vi "gjson_UnFlatten.vi"(6 "UnFlattenedData In":string, 8 "error in":errorcluster, 10 "Variant":variant, 11 "JSON String In":string) -> (0 "error out":errorcluster, 2 "UnFlattenData Out":string, 3 "JSON String Out":string)   [LabVIEW 2015, in "Json2Labv.lvlib"]
uses:
  Json2Labv.lvlib
  <vilib>/regexp/Match Regular Expression.xnode
  <vilib>/Utility/VariantDataType/VariantType.lvlib
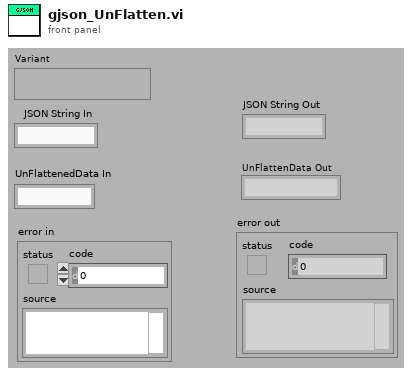
[diagram p1: front panel]
types:
  T1 = typedef "VariantType.lvlib/Type.ctl" = enum8{"Invalid Type", "Void", "I8", "I16", "I32", "I64", "U8", "U16", "U32", "U64", "Single Float", "Double Float", "Extended Float", "Single Complex", "Double Complex", "Extended Complex", "Enum U8", "Enum U16", "Enum U32", "Enum U64", "Single Float With Unit", "Double Float With Unit", "Extended Float With Unit", "Single Complex with Unit", "Double Complex with Unit", "Extended Complex with Unit", "Boolean", "String", "Path", "Picture", "Tag", "Array", "Cluster", "Variant", "LV Variant", "Waveform", "Timestamp", "Digital Waveform", "Digital Data", "ExpressData", "Refnum", "External Data", "VI", "Poly VI", "LabVIEW Class Instance", "Fixed Point"}
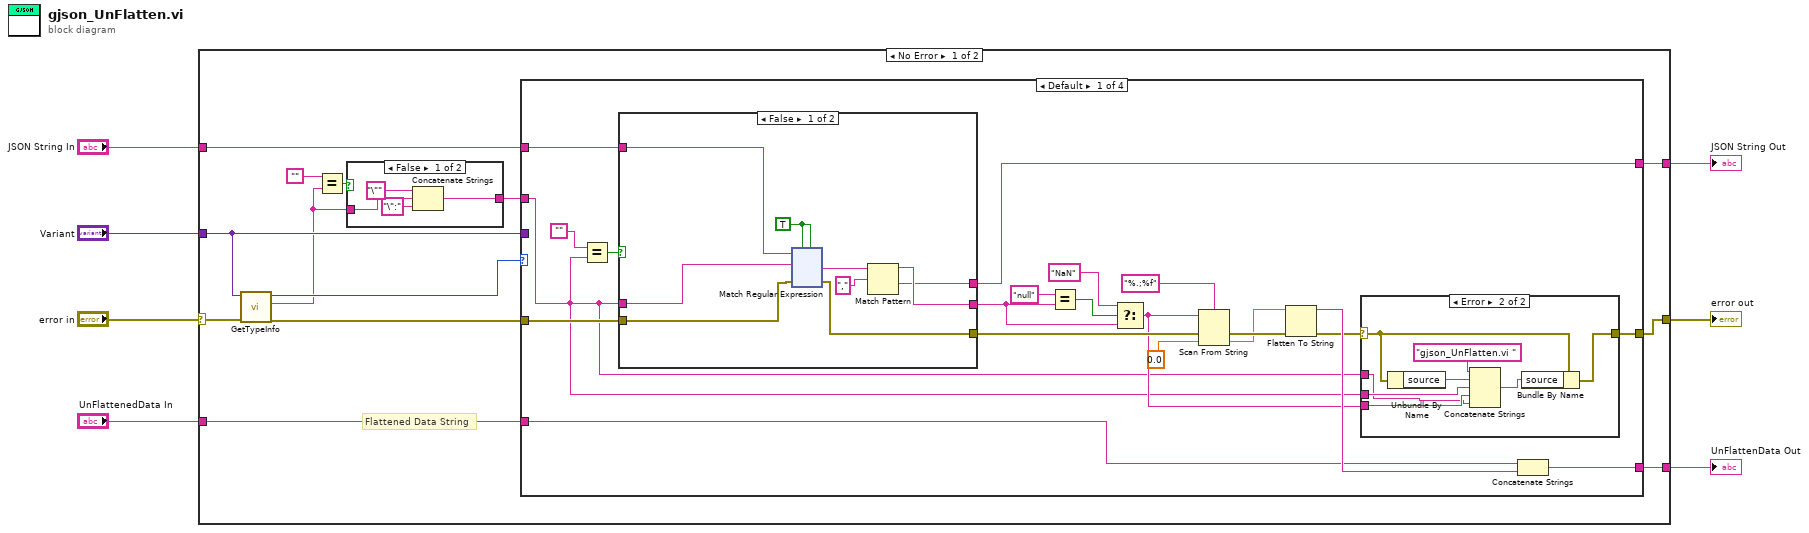
[diagram p0: block diagram]
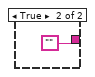
[diagram p2: hidden frame]
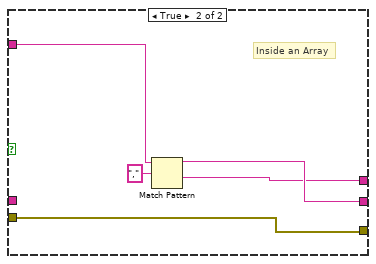
[diagram p4: hidden frame]
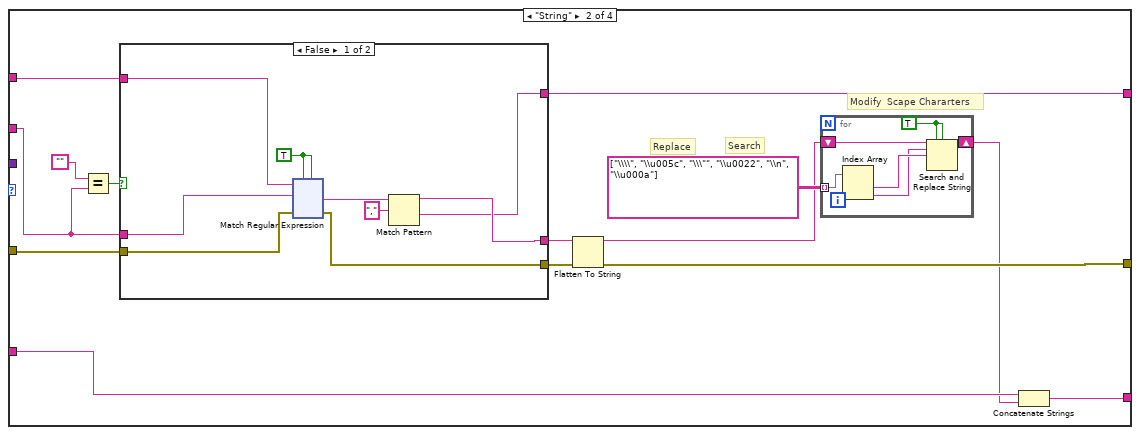
[diagram p5: hidden frame]
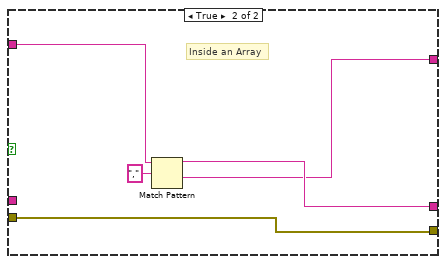
[diagram p6: hidden frame]
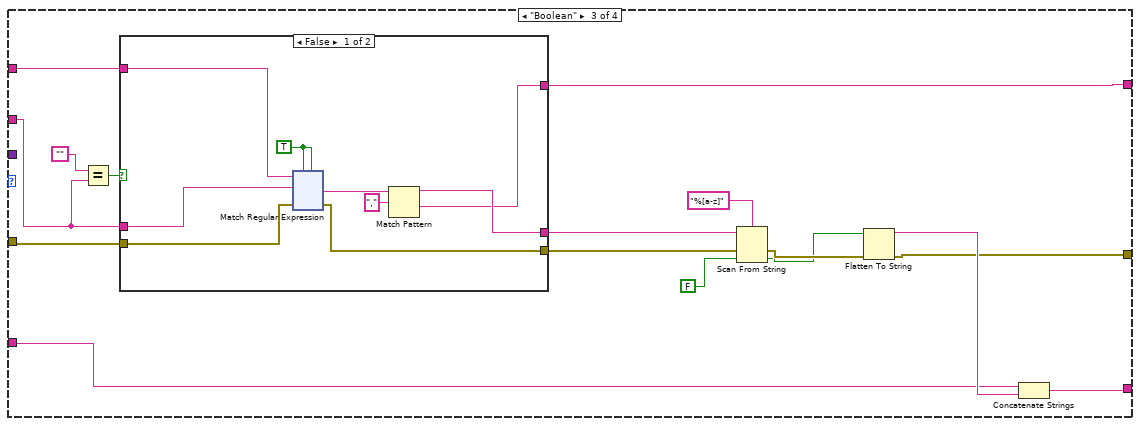
[diagram p7: hidden frame]
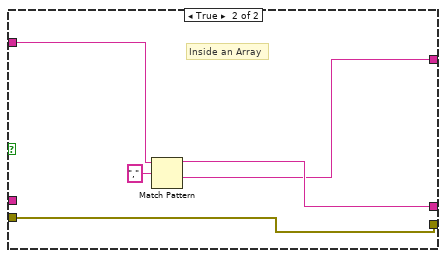
[diagram p8: hidden frame]
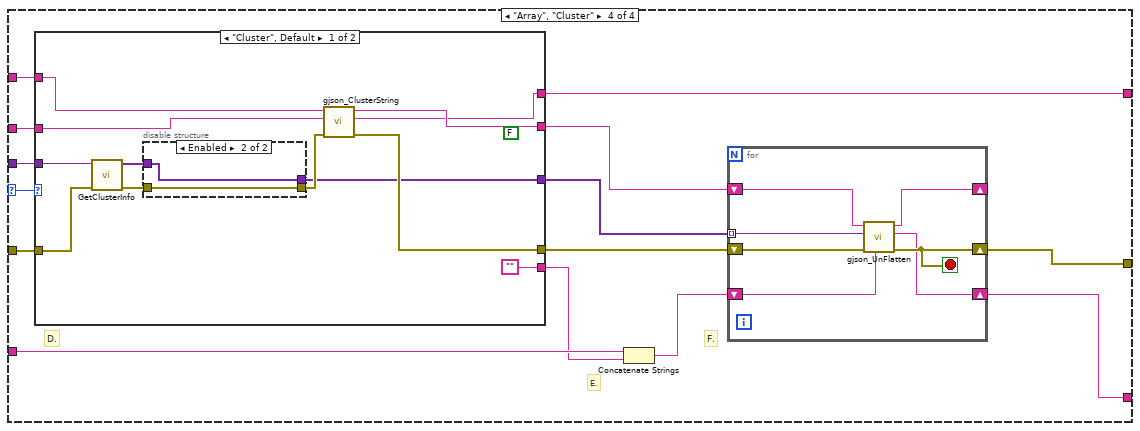
[diagram p9: hidden frame]
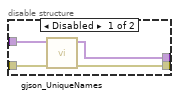
[diagram p10: hidden frame]
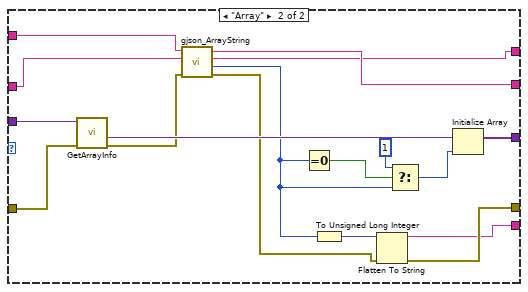
[diagram p11: hidden frame]
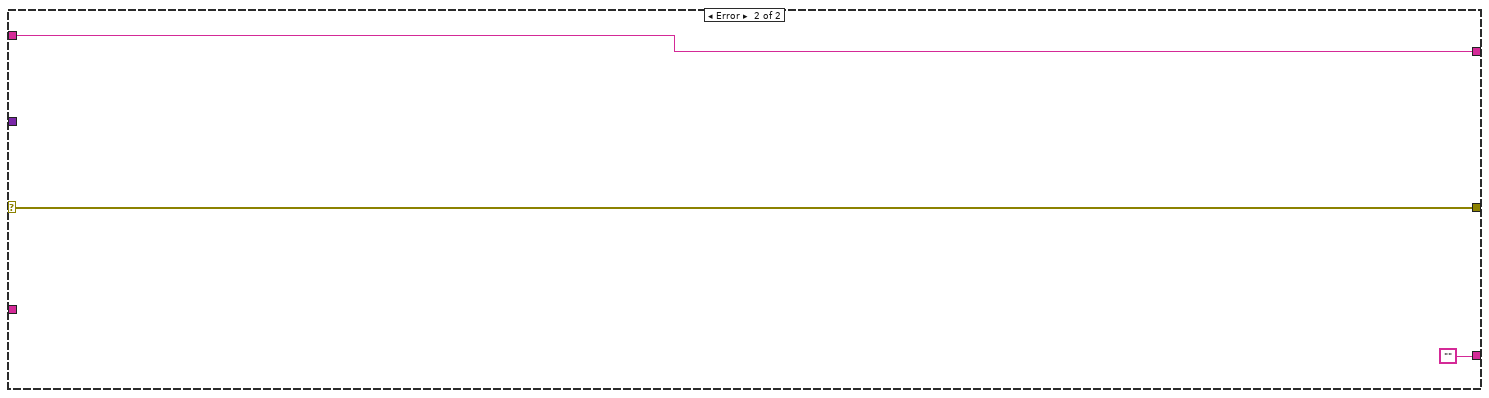
[diagram p12: hidden frame]
diagram:
  n1 = case shown="No Error" "error in" {
    selector: "error in" -> [w18 w525]
    tunnel: [w20 w525] -> w7
    tunnel: [w19 w524] -> w5
    tunnel: "JSON String In" -> [w13 w524]
    tunnel: "Variant" -> [w16 _]
    tunnel: "UnFlattenedData In" -> [w15 _]
    tunnel: [w12 ""] -> w4
    frame No Error {
      # "Flattened Data String"
      n2 = call <vilib>:"GetTypeInfo.vi"("error in (no error)"=w18, "Variant"=w16) -> ("error out"=w14:errorcluster, "Name"=w10:string, "Type Enum"=w17:T1)  [unwired: 5 in, 2 out]
      n3 = Equal?(x="", y=w10) -> (x = y?=w8:bool)
      n4 = case shown="False" w8 {
        tunnel: w10 -> [w24 _]
        tunnel: [w21 ""] -> w9
        frame False {
          n5 = Concatenate Strings("\"" ("string"), w24, "\":" ("string")) -> (w21:string)
        }
        frame True {
        }
      }
      n6 = case shown="Default" w17 {
        selector: w17 -> [_ _ _ w476]
        tunnel: w16 -> [_ _ _ w480]
        tunnel: w14 -> [w45 w191 w337 w479]
        tunnel: [w40 w189 w333 w470] -> w19
        tunnel: [w33 w184 w332 w475] -> w20
        tunnel: w13 -> [w46 w192 w338 w474]
        tunnel: w15 -> [w35 w186 w336 w469]
        tunnel: [w38 w185 w335 w472] -> w12
        tunnel: w9 -> [w26 w190 w334 w471]
        frame Default {
          n7 = Equal?(x="", y=w26) -> (x = y?=w37:bool)
          n8 = case shown="False" w37 {
            tunnel: w26 -> [w57 _]
            tunnel: w46 -> [w63 w180]
            tunnel: w45 -> [w62 w176]
            tunnel: [w61 w176] -> w41
            tunnel: [w58 w177] -> w40
            tunnel: [w59 w178] -> w29
            frame False {
              w64 = TRUE ("ignore case? (F)")
              n9 = xnode "Match Regular Expression"("input string"=w63, "regular expression"=w57, "error in"=w62, "ignore case? (F)"=w64, "multiline? (F)"=w64) -> ("after match"=w56:string, "error out"=w61:errorcluster)  [unwired: 1 in, 3 out]
              n10 = Match Pattern(string=w56, regular expression=",") -> (before substring=w59:string, after substring=w58:string)  [unwired: 1 in, 2 out]
            }
            frame True {
              # "Inside an Array"
              n11 = Match Pattern(string=w180, regular expression=",") -> (before substring=w178:string, after substring=w177:string)  [unwired: 1 in, 2 out]
            }
          }
          n12 = Equal?(x="null", y=w29) -> (x = y?=w30:bool)
          n13 = Select(t="NaN", s=w30, f=w29) -> (s? t:f=w27:string)
          n14 = Scan From String(format string="%.;%f", input string=w27, error in=w41, default 1=0.0) -> (error out=w43:errorcluster, output 1=w42:dbl)  [unwired: 1 in, 2 out]
          n15 = Flatten To String(anything=w42, error in (no error)=w43) -> (data string=w39:string, error out=w34:errorcluster)  [unwired: 2 in, 1 out]
          n16 = case shown="Error" w34 {
            selector: w34 -> [w47 w52]
            tunnel: [w47 w51] -> w33
            tunnel: w26 -> [_ w50]
            tunnel: w27 -> [_ w49]
            tunnel: w26 -> [_ w48]
            frame No Error {
            }
            frame Error {
              n17 = Unbundle By Name(w52) -> ("source"=w55:string)
              n18 = Concatenate Strings("gjson_UnFlatten.vi ", w55, w50, w49, w48) -> (w53:string)
              n19 = Bundle By Name(cluster=w52, "source"=w53) -> (w51:errorcluster)
            }
          }
          n20 = Concatenate Strings(w35, w39) -> (w38:string)
        }
        frame "String" {
          # "Replace"
          # "Search"
          # "Modify  Scape Chararters"
          n21 = Equal?(x="", y=w190) -> (x = y?=w194:bool)
          n22 = case shown="False" w194 {
            tunnel: w190 -> [w205 _]
            tunnel: w192 -> [w208 w325]
            tunnel: w191 -> [w207 w321]
            tunnel: [w206 w321] -> w188
            tunnel: [w201 w322] -> w189
            tunnel: [w202 w323] -> w187
            frame False {
              w209 = TRUE ("ignore case? (F)")
              n23 = xnode "Match Regular Expression"("input string"=w208, "regular expression"=w205, "error in"=w207, "ignore case? (F)"=w209, "multiline? (F)"=w209) -> ("after match"=w204:string, "error out"=w206:errorcluster)  [unwired: 1 in, 3 out]
              n24 = Match Pattern(string=w204, regular expression=",") -> (before substring=w202:string, after substring=w201:string)  [unwired: 1 in, 2 out]
            }
            frame True {
              # "Inside an Array"
              n25 = Match Pattern(string=w325, regular expression=",") -> (before substring=w323:string, after substring=w322:string)  [unwired: 1 in, 2 out]
            }
          }
          n26 = Flatten To String(anything=w187, error in (no error)=w188) -> (data string=w181:string, error out=w184:errorcluster)  [unwired: 2 in, 1 out]
          n27 = for {
            shift-right: [w199] -> w182
            shift-left: w181 -> [w200]
            tunnel: string[][] [["\\\\", "\\u005c"], ["\\\"", "\\u0022"], ["\\n", "\\u000a"]] -> [w198] mode=indexing
            w197 = TRUE ("replace all? (F)")
            n28 = Index Array(array=w198) -> (element #1=w196:string, element #2=w195:string)  [unwired: 2 in]
            n29 = Search and Replace String(replace all?=w197, case sensitive?=w197, input string=w200, search string=w195, replace string=w196) -> (result string=w199:string)  [unwired: 3 in, 3 out]
          }
          n30 = Concatenate Strings(w186, w182) -> (w185:string)
        }
        frame "Boolean" {
          n31 = Equal?(x="", y=w334) -> (x = y?=w340:bool)
          n32 = case shown="False" w340 {
            tunnel: w334 -> [w346 _]
            tunnel: w338 -> [w349 w466]
            tunnel: w337 -> [w348 w462]
            tunnel: [w347 w462] -> w328
            tunnel: [w342 w463] -> w333
            tunnel: [w343 w464] -> w331
            frame False {
              w350 = TRUE ("ignore case? (F)")
              n33 = xnode "Match Regular Expression"("input string"=w349, "regular expression"=w346, "error in"=w348, "ignore case? (F)"=w350, "multiline? (F)"=w350) -> ("after match"=w345:string, "error out"=w347:errorcluster)  [unwired: 1 in, 3 out]
              n34 = Match Pattern(string=w345, regular expression=",") -> (before substring=w343:string, after substring=w342:string)  [unwired: 1 in, 2 out]
            }
            frame True {
              # "Inside an Array"
              n35 = Match Pattern(string=w466, regular expression=",") -> (before substring=w464:string, after substring=w463:string)  [unwired: 1 in, 2 out]
            }
          }
          n36 = Scan From String(format string="%[a-z]", input string=w331, error in=w328, default 1=FALSE) -> (error out=w330:errorcluster, output 1=w327:bool)  [unwired: 1 in, 2 out]
          n37 = Flatten To String(anything=w327, error in (no error)=w330) -> (data string=w341:string, error out=w332:errorcluster)  [unwired: 2 in, 1 out]
          n38 = Concatenate Strings(w336, w341) -> (w335:string)
        }
        frame "Array", "Cluster" {
          # "E."
          # "F."
          # "D."
          n39 = case shown="\"Cluster\", Default" w476 {
            tunnel: w480 -> [w491 w508]
            tunnel: w479 -> [w492 w512]
            tunnel: [w481 w515] -> w478
            tunnel: [w486 w510] -> w477
            tunnel: w474 -> [w489 w500]
            tunnel: [w488 w507] -> w473
            tunnel: w471 -> [w484 w499]
            tunnel: [w485 w506] -> w470
            tunnel: ["" w504] -> w467
            frame "Cluster", Default {
              (unwired) FALSE
              n40 = call <vilib>:"GetClusterInfo.vi"("error in (no error)"=w492, "Variant"=w491) -> ("error out"=w490:errorcluster, "Cluster Elements"=w482:variant[])  [unwired: 8 in]
              n41 = disable-structure shown="Enabled" {
                disable-tunnel: w490 -> [w496 w497]
                disable-tunnel: [w495 w497] -> w487
                disable-tunnel: w482 -> [w494 w498]
                disable-tunnel: [w493 w498] -> w481
                frame Disabled {
                  n42 = call "gjson_UniqueNames.vi"("error in"=w496, "Cluster Elements"=w494) -> ("error out"=w495:errorcluster, "Cluster Elements Out"=w493:variant[])  [unwired: 8 in]
                }
                frame Enabled {
                }
              }
              n43 = call "gjson_ClusterString.vi"("error in"=w487, "Cluster to Find"=w484, "String In"=w489) -> ("error out"=w486:errorcluster, "Rest"=w485:string, "Cluster"=w488:string)  [unwired: 6 in]
            }
            frame "Array" {
              n44 = call <vilib>:"GetArrayInfo.vi"("error in (no error)"=w512, "Variant"=w508) -> ("error out"=w502:errorcluster, "ArrayElement"=w509:variant)  [unwired: 6 in, 2 out]
              n45 = call "gjson_ArrayString.vi"("error in"=w502, "Array to Find"=w499, "String In"=w500) -> ("error out"=w501:errorcluster, "ArraySize"=w503:i32, "Rest"=w506:string, "Array"=w507:string)  [unwired: 5 in]
              n46 = Equal To 0?(x=w503) -> (x = 0?=w514:bool)
              n47 = To Unsigned Long Integer(number=w503) -> (unsigned 32bit integer=w511:u32)
              n48 = Flatten To String(anything=w511, error in (no error)=w501) -> (data string=w504:string, error out=w510:errorcluster)  [unwired: 2 in, 1 out]
              n49 = Select(t=1, s=w514, f=w503) -> (s? t:f=w505:i32)
              n50 = Initialize Array(w509, w505) -> (w515:variant[])
            }
          }
          n51 = Concatenate Strings(w469, w467) -> (w468:string)
          n52 = for {
            shift-right: [w519] -> _
            shift-left: w473 -> [w520]
            tunnel: w478 -> [w516] mode=indexing
            shift-right: [w522] -> w475
            shift-left: w477 -> [w521]
            shift-right: [w517] -> w472
            shift-left: w468 -> [w518]
            stop <- w522 stop-if-true
            n53 = call "gjson_UnFlatten.vi"("UnFlattenedData In"=w518, "error in"=w521, "Variant"=w516, "JSON String In"=w520) -> ("error out"=w522:errorcluster, "UnFlattenData Out"=w517:string, "JSON String Out"=w519:string)  [unwired: 5 in]
          }
        }
      }
    }
    frame Error {
    }
  }
  "error out" <- w7
  "JSON String Out" <- w5
  "UnFlattenData Out" <- w4
